vi "Write Data.vi"(0 "Bit In (SCLK & SYNC)":bool, 7 "Word In (DIN)":u32, 11 "error in (no error)":errorcluster, 12 "Socket Mask":u32, 13 "Line":T1) -> (15 "error out":errorcluster)   [LabVIEW 2017, in "FPGA-SRL.lvlib"]
uses:
  FPGA-SRL.lvlib
  Type Defs/Write Line Enum.ctl
  <vilib>/rvi/eio/common/nirviEmuTemplateMethod_errors.vi
  <vilib>/eio/EIONode/EIONode.xnode
  Debug Global.vi
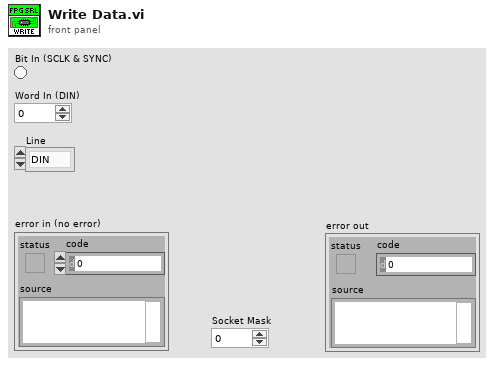
[diagram p1: front panel]
types:
  T1 = typedef "FPGA-SRL.lvlib/Write Line Enum.ctl" = enum16{"DIN", "SYNC", "SCLK"}
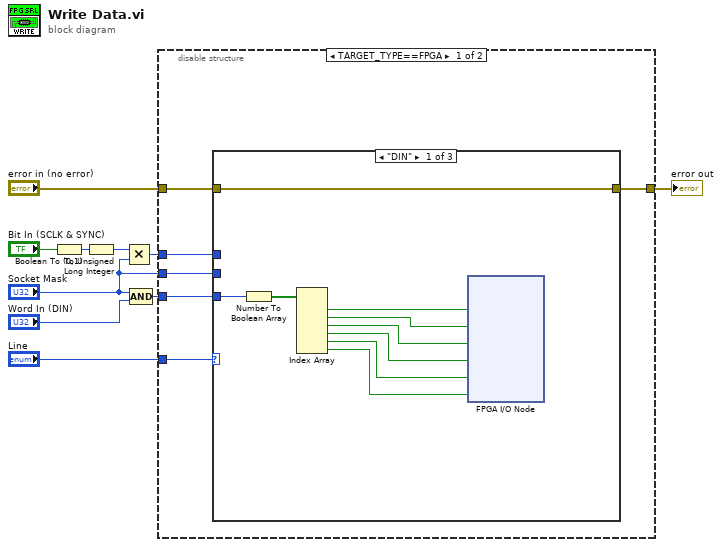
[diagram p0: block diagram]
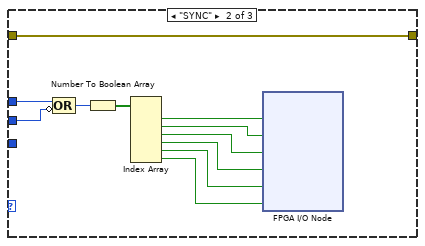
[diagram p2: hidden frame]
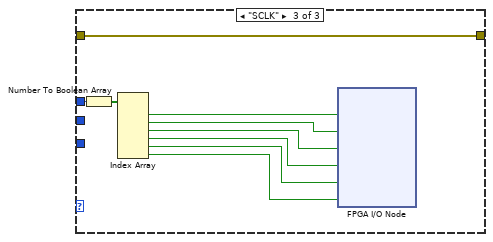
[diagram p3: hidden frame]
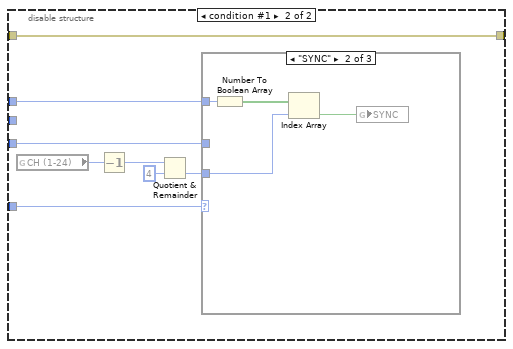
[diagram p4: hidden frame]
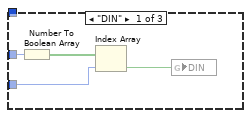
[diagram p5: hidden frame]
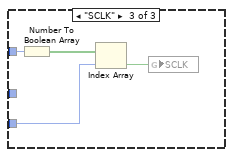
[diagram p6: hidden frame]
diagram:
  n1 = Boolean To (0,1)(Boolean="Bit In (SCLK & SYNC)") -> (0, 1=w4:i16)
  n2 = To Unsigned Long Integer(number=w4) -> (unsigned 32bit integer=w3:u32)
  n3 = Multiply(x=w3, y="Socket Mask") -> (x*y=w2:u32)
  n4 = Compound Arithmetic op=AND("Socket Mask", "Word In (DIN)") -> (w6:u32)
  n5 = disable-structure shown="TARGET_TYPE==FPGA" {
    disable-tunnel: "Line" -> [w16 w53]
    disable-tunnel: [w15 w52] -> w9
    disable-tunnel: "error in (no error)" -> [w14 w52]
    disable-tunnel: w6 -> [w13 w51]
    disable-tunnel: w2 -> [w12 w50]
    disable-tunnel: "Socket Mask" -> [w11 _]
    frame condition #0 (active) {
      n6 = case shown="\"DIN\"" w16 {
        tunnel: [w25 w36 w43] -> w15
        tunnel: w14 -> [w25 w36 w43]
        tunnel: w13 -> [w23 _ _]
        tunnel: w12 -> [_ w28 w44]
        tunnel: w11 -> [_ w27 _]
        frame "DIN" {
          n7 = Number To Boolean Array(number=w23) -> (Boolean array=w24:bool[])
          n8 = Index Array(array=w24) -> (element #1=w22:bool, element #2=w21:bool, element #3=w20:bool, element #4=w19:bool, element #5=w18:bool, element #6=w17:bool)  [unwired: 6 in]
          n9 = xnode "FPGA I/O Node"("DIN_1"=w22, "DIN_2"=w21, "DIN_3"=w20, "DIN_4"=w19, "DIN_5"=w18, "DIN_6"=w17) -> ()  [unwired: 7 in, 7 out]
        }
        frame "SYNC" {
          n10 = Compound Arithmetic op=OR(w28, invert w27) -> (w26:u32)
          n11 = Number To Boolean Array(number=w26) -> (Boolean array=w35:bool[])
          n12 = Index Array(array=w35) -> (element #1=w34:bool, element #2=w33:bool, element #3=w32:bool, element #4=w31:bool, element #5=w30:bool, element #6=w29:bool)  [unwired: 6 in]
          n13 = xnode "FPGA I/O Node"("SYNC_1"=w34, "SYNC_2"=w33, "SYNC_3"=w32, "SYNC_4"=w31, "SYNC_5"=w30, "SYNC_6"=w29) -> ()  [unwired: 6 in, 6 out]
        }
        frame "SCLK" {
          n14 = Number To Boolean Array(number=w44) -> (Boolean array=w45:bool[])
          n15 = Index Array(array=w45) -> (element #1=w42:bool, element #2=w41:bool, element #3=w40:bool, element #4=w39:bool, element #5=w38:bool, element #6=w37:bool)  [unwired: 6 in]
          n16 = xnode "FPGA I/O Node"("SCLK_1"=w42, "SCLK_2"=w41, "SCLK_3"=w40, "SCLK_4"=w39, "SCLK_5"=w38, "SCLK_6"=w37) -> ()  [unwired: 6 in, 6 out]
        }
      }
    }
    frame condition #1 {
      n17 = global read "Debug Global.vi" "CH (1-24)"() -> (w49:i32)
      n18 = Decrement(x=w49) -> (x-1=w46:i32)
      n19 = Quotient & Remainder(x=w46, y=4) -> (floor(x/y)=w47:i32)  [unwired: 1 out]
      n20 = case shown="\"SYNC\"" w53 {
        tunnel: w51 -> [w55 _ _]
        tunnel: w47 -> [w54 w58 w62]
        tunnel: w50 -> [_ w59 w63]
        frame "DIN" {
          n21 = Number To Boolean Array(number=w55) -> (Boolean array=w57:bool[])
          n22 = Index Array(array=w57, index=w54) -> (element=w56:bool)
          n23 = global write "Debug Global.vi" "DIN"(w56) -> ()
        }
        frame "SYNC" {
          n24 = Number To Boolean Array(number=w59) -> (Boolean array=w61:bool[])
          n25 = Index Array(array=w61, index=w58) -> (element=w60:bool)
          n26 = global write "Debug Global.vi" "SYNC"(w60) -> ()
        }
        frame "SCLK" {
          n27 = Number To Boolean Array(number=w63) -> (Boolean array=w65:bool[])
          n28 = Index Array(array=w65, index=w62) -> (element=w64:bool)
          n29 = global write "Debug Global.vi" "SCLK"(w64) -> ()
        }
      }
    }
  }
  "error out" <- w9
